vi "Dictionary to Chart.vi"(8 "error in (no error)":errorcluster, 10 "Display":T1=enum."R and Theta" caption="Enum", 11 "Results.Results (Dictionary)":cluster{"key":string, "value":dbl}[](array[cluster])) -> (0 "error out":errorcluster, 1 "XY Graph":cluster{dbl[], dbl[]}[](array[cluster]), 2 "Y/Theta Array":waveform(dbl)[](array[waveform]), 3 "X/R Array":waveform(dbl)[](array[waveform]), 4 "Plot Names":string[](array[string]))   [LabVIEW 2016, in "Instrument.Lockin.lvclass"]
uses:
  Instrument.Lockin.lvclass
  Instrument.Lockinl.UI/Typedefs/Display-Enum.ctl
  Typedefs/Results Type--Enum.ctl
  Instrument.Lockinl.UI/Instrument.Lockin.UI.lvclass
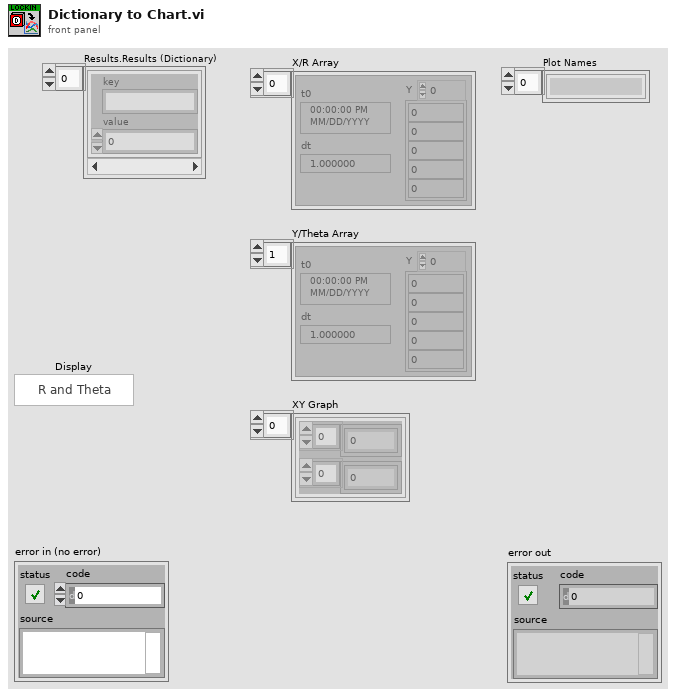
[diagram p1: front panel]
types:
  T1 = typedef "Instrument.Lockin.UI.lvclass/Display-Enum.ctl" = enum16{"X and Y", "R and Theta", "Mean"}
  T2 = typedef "Instrument.Lockin.lvclass/Results Type--Enum.ctl" = enum16{"X", "Y", "R", "Theta", "Mean"}
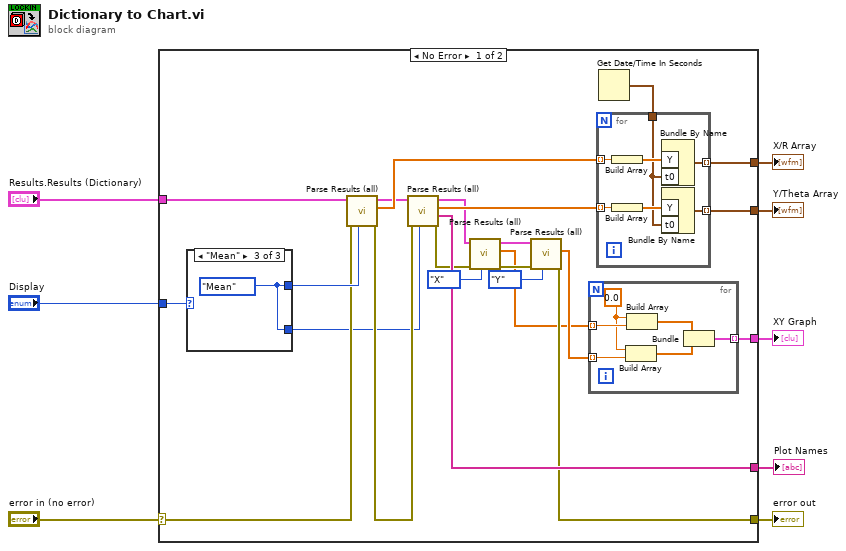
[diagram p0: block diagram]
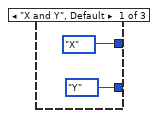
[diagram p2: hidden frame]
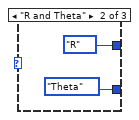
[diagram p3: hidden frame]
diagram:
  n1 = case shown="No Error" "error in (no error)" {
    selector: "error in (no error)" -> [w22 w50]
    tunnel: [w31 _] -> w8
    tunnel: [w30 _] -> w7
    tunnel: "Display" -> [w29 _]
    tunnel: "Results.Results (Dictionary)" -> [w26 _]
    tunnel: [w13 w50] -> w3
    tunnel: [w27 _] -> w2
    tunnel: [w20 _] -> w1
    frame No Error {
      n2 = case shown="\"Mean\"" w29 {
        tunnel: [Results_Type--Enum."X" ("Type") Results_Type--Enum."R" ("Type") w36] -> w23
        tunnel: [Results_Type--Enum."Y" ("Type") Results_Type--Enum."Theta" ("Type") w36] -> w19
        frame "X and Y", Default {
        }
        frame "R and Theta" {
        }
        frame "Mean" {
          w36 = Results_Type--Enum."Mean" ("Type")
        }
      }
      n3 = call "Parse Results (all).vi"("Type"=w23, "error in (no error)"=w22, "Results (Dictionary)"=w26) -> ("error out"=w21:errorcluster, "Data"=w25:dbl[], "Results (Dictionary)"=w24:cluster{"key":string, "value":dbl}[])  [unwired: 5 in, 1 out]
      n4 = call "Parse Results (all).vi"("Type"=w19, "error in (no error)"=w21, "Results (Dictionary)"=w24) -> ("error out"=w14:errorcluster, "Names"=w20:string[], "Data"=w18:dbl[], "Results (Dictionary)"=w16:cluster{"key":string, "value":dbl}[])  [unwired: 5 in]
      n5 = call "Parse Results (all).vi"("Type"=Results_Type--Enum."X", "error in (no error)"=w14, "Results (Dictionary)"=w16) -> ("error out"=w15:errorcluster, "Data"=w9:dbl[], "Results (Dictionary)"=w17:cluster{"key":string, "value":dbl}[])  [unwired: 5 in, 1 out]
      n6 = call "Parse Results (all).vi"("Type"=Results_Type--Enum."Y", "error in (no error)"=w15, "Results (Dictionary)"=w17) -> ("error out"=w13:errorcluster, "Data"=w10:dbl[])  [unwired: 5 in, 2 out]
      n7 = for {
        tunnel: w9 -> [w42] mode=indexing
        tunnel: w10 -> [w41] mode=indexing
        tunnel: [w37] -> w27 mode=indexing
        w40 = 0.0
        n8 = Build Array(w40, w41) -> (w38:dbl[])
        n9 = Build Array(w40, w42) -> (w39:dbl[])
        n10 = Bundle(w39, w38) -> (w37:cluster{dbl[], dbl[]})  [unwired: 1 in]
      }
      n11 = Get Date/Time In Seconds() -> (seconds since 1Jan1904=w28:timestamp)
      n12 = for {
        tunnel: w25 -> [w49] mode=indexing
        tunnel: w18 -> [w43] mode=indexing
        tunnel: [w48] -> w30 mode=indexing
        tunnel: [w47] -> w31 mode=indexing
        tunnel: w28 -> [w44]
        tunnel: [w43] -> _ mode=indexing
        n13 = Build Array(w49) -> (w46:dbl[])
        n14 = Build Array(w43) -> (w45:dbl[])
        n15 = Bundle By Name("Y"=w46, "t0"=w44) -> (w48:waveform(dbl))  [unwired: 1 in]
        n16 = Bundle By Name("Y"=w45, "t0"=w44) -> (w47:waveform(dbl))  [unwired: 1 in]
      }
    }
    frame Error {
    }
  }
  "Y/Theta Array" <- w8
  "X/R Array" <- w7
  "error out" <- w3
  "XY Graph" <- w2
  "Plot Names" <- w1
